vi "KBRD Query Till Position v2 (SubVI).vi"(11 "Queue in":refnum<queue>) -> (3 "Queue out":refnum<queue>)   [LabVIEW 2018]
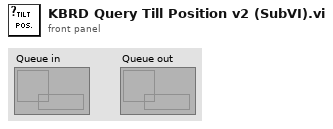
[diagram p1: front panel]
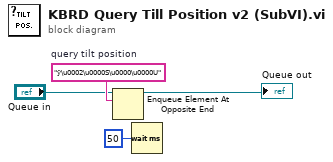
[diagram p0: block diagram]
diagram:
  w3 = "ÿ\u0002\u0000S\u0000\u0000U"  # query tilt position
  n1 = Enqueue Element At Opposite End(queue="Queue in", element=w3) -> (queue out=→"Queue out":refnum<queue>)  [unwired: 2 in, 2 out]
  n2 = Wait (ms)(milliseconds to wait=u32 50) -> ()  [unwired: 1 out]
